vi "putFile.vi"(7 "isDir?":bool, 8 "error in (no error)":errorcluster, 9 "local path":path, 10 "remote path":string, 11 "ConnectionData":T1) -> (0 "error out":errorcluster, 3 "local path out":path)   [LabVIEW 2016]
uses:
  connectionData.ctl
panel:
  # "Puts a file to a remote location. Uses the pscp utility to perform the\ntransfer. This VI expects to find pscp.exe in the same dirctory that\nthis VI is located in.\nDOWNLOAD: http://www.chiark.greenend.org.uk/~sgtatham/putty/download.html"
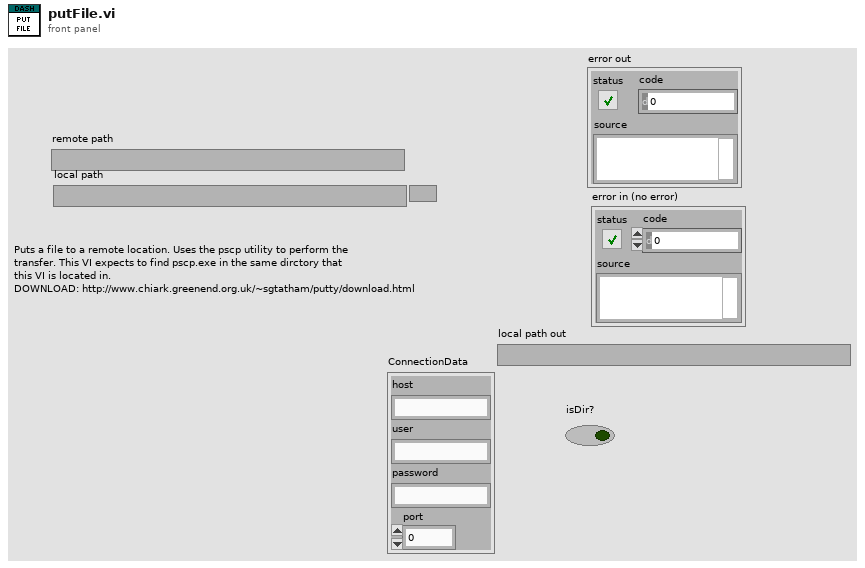
[diagram p1: front panel]
types:
  T1 = typedef "connectionData.ctl" = cluster{"host":string, "user":string, "password":string, "port":u16}
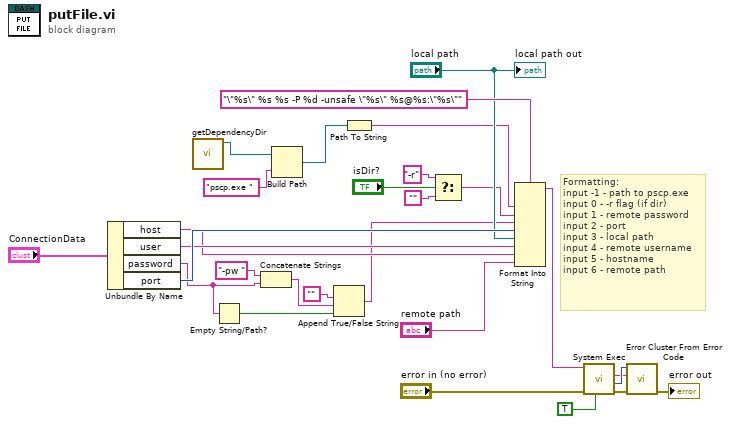
[diagram p0: block diagram]
diagram:
  # "Formatting:\ninput -1 - path to pscp.exe\ninput 0 - -r flag (if dir)\ninput 1 - remote password\ninput 2 - port\ninput 3 - local path\ninput 4 - remote username\ninput 5 - hostname\ninput 6 - remote path"
  n1 = Unbundle By Name("ConnectionData") -> ("host"=w17:string, "user"=w18:string, "password"=w7:string, "port"=w20:u16)
  n2 = call "getDependencyDir.vi"() -> ("Dependency Directory"=w3:path)  [unwired: 11 in]
  n3 = Empty String/Path?(string/path=w7) -> (empty?=w10:bool)
  n4 = Concatenate Strings("-pw " ("string"), w7) -> (w8:string)
  n5 = Build Path(base path=w3, name or relative path="pscp.exe ") -> (appended path=w2:path)
  n6 = Append True/False String(1:w10, 2:w8, 3:"") -> (0:w5:string)  [unwired: 1 in]
  n7 = Path To String(path=w2) -> (string=w1:string)
  n8 = Select(t="-r" ("string"), s="isDir?", f="") -> (s? t:f=w11:string)
  n9 = Format Into String(format string="\"%s\" %s %s -P %d -unsafe \"%s\" %s@%s:\"%s\"", w1, w11, w5, w20, "local path", w18, w17, "remote path") -> (resulting string=w15:string)  [unwired: 2 in, 1 out]
  n10 = call <vilib>:"System Exec.vi"("run minimized? (F)"=TRUE, "error in (no error)"="error in (no error)", "command line"=w15) -> ("error out"=w22:errorcluster, "return code"=w26:i32, "standard error"=w25:string)  [unwired: 5 in, 1 out]
  n11 = call <vilib>:"Error Cluster From Error Code.vi"("error in (no error)"=w22, "error message (\"\")"=w25, "error code (0)"=w26) -> ("error out"=→"error out":errorcluster)  [unwired: 6 in]
  "local path out" <- "local path"
